vi "NEAR_IR_NM_to_FAR_IR_CM.vi"(11 "Near IR / nm":dbl format="%#_6f") -> (3 "Far IR / cm-1":dbl)   [LabVIEW 2020]
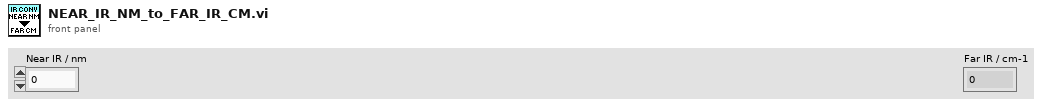
[diagram p1: front panel]
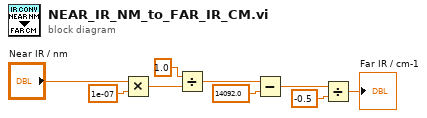
[diagram p0: block diagram]
diagram:
  n1 = Multiply(x="Near IR / nm", y=1e-07) -> (x*y=w7:dbl)
  n2 = Divide(x=1.0, y=w7) -> (x/y=w5:dbl)
  n3 = Subtract(x=w5, y=14092.0) -> (x-y=w3:dbl)
  n4 = Divide(x=w3, y=-0.5) -> (x/y=→"Far IR / cm-1":dbl)
